vi "ellipse model easy.vi"(3 "output control":T1, 4 "data":variant, 5 "X":dbl[](array[numeric]), 6 "a":dbl[](array[numeric])) -> (0 "error out":errorcluster, 1 "f'(X,a)":dbl[][](array[numeric]), 2 "f(X,a)":dbl[](array[numeric]))   [LabVIEW 2013]
doc: "Implements an ellipse model function to be passed to the Nonlinear Curve Fit.vi."
uses:
  <vilib>/gmath/NumericalOptimization/LM_output select.ctl
  <vilib>/gmath/NI_Gmath.lvlib
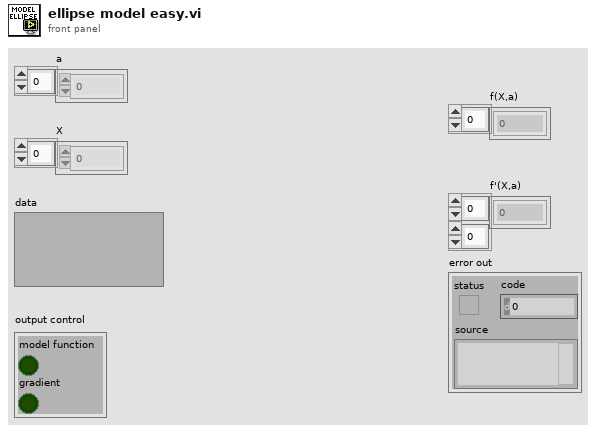
[diagram p1: front panel]
types:
  T1 = typedef "NI_Gmath.lvlib/LM_output select.ctl" = cluster{"model function":bool, "gradient":bool}
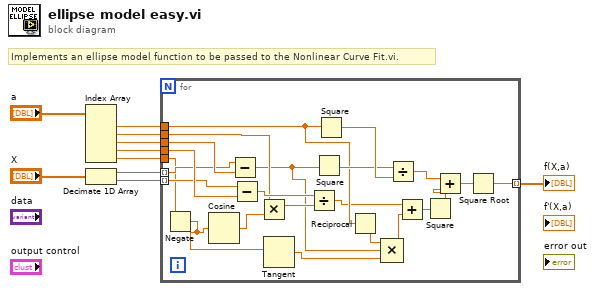
[diagram p0: block diagram]
diagram:
  # "Implements an ellipse model function to be passed to the Nonlinear Curve Fit.vi."
  n1 = Index Array(array="a") -> (element #1=w8:dbl, element #2=w7:dbl, element #3=w6:dbl, element #4=w2:dbl, element #5=w1:dbl)  [unwired: 5 in]
  n2 = Decimate 1D Array("X") -> (w4:dbl[], w3:dbl[])
  n3 = for {
    tunnel: w4 -> [w13] mode=indexing
    tunnel: w8 -> [w23]
    tunnel: w7 -> [w26]
    tunnel: w6 -> [w14]
    tunnel: [w32] -> w5 mode=indexing
    tunnel: w3 -> [w15] mode=indexing
    tunnel: w2 -> [w16]
    tunnel: w1 -> [w12]
    n4 = Negate(x=w12) -> (-x=w11:dbl)
    n5 = Cosine(x=w11) -> (cos(x)=w25:dbl)
    n6 = Subtract(x=w13, y=w14) -> (x-y=w24:dbl)
    n7 = Subtract(x=w15, y=w16) -> (x-y=w28:dbl)
    n8 = Multiply(x=w26, y=w25) -> (x*y=w27:dbl)
    n9 = Tangent(1:w11) -> (0:w17:dbl)
    n10 = Divide(x=w28, y=w27) -> (x/y=w21:dbl)
    n11 = Square(x=w24) -> (x^2=w29:dbl)
    n12 = Square(x=w23) -> (x^2=w31:dbl)
    n13 = Reciprocal(x=w23) -> (1/x=w22:dbl)
    n14 = Compound Arithmetic op=MULTIPLY(w22, w24, w17) -> (w20:dbl)
    n15 = Divide(x=w29, y=w31) -> (x/y=w30:dbl)
    n16 = Add(x=w21, y=w20) -> (x+y=w19:dbl)
    n17 = Square(x=w19) -> (x^2=w18:dbl)
    n18 = Add(x=w30, y=w18) -> (x+y=w33:dbl)
    n19 = Square Root(x=w33) -> (sqrt(x)=w32:dbl)
  }
  "f(X,a)" <- w5
